vi "Init_Stimulus.vi"   [LabVIEW 2015]
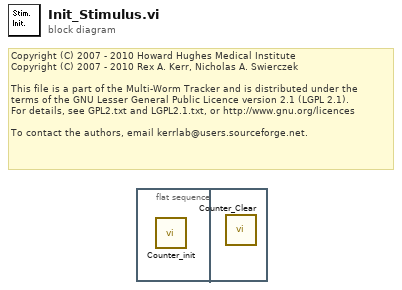
[diagram p0: block diagram]
diagram:
  # "Copyright (C) 2007 - 2010 Howard Hughes Medical Institute\nCopyright (C) 2007 - 2010 Rex A. Kerr, Nicholas A. Swierczek\n \nThis file is a part of the Multi-Worm Tracker and is distributed under the\nterms of the GNU Lesser General Public Licence version 2.1 (LGPL 2.1).\nFor details, see GPL2.txt and LGPL2.1.txt, or http://www.gnu.org/licences\n \nTo contact the authors, email kerrlab@users.sourceforge.net."
  n1 = flat-sequence {
    frame #0 {
      n2 = call "Counter_init.vi"() -> ()  [unwired: 1 out]
    }
    frame #1 {
      n3 = call "Counter_Clear.vi"() -> ()  [unwired: 1 out]
    }
  }
